vi "AmsRouterNotification Event Callback.vi"(4 "User Parameter":refnum<user-event>, 5 "Event Data":cluster{"sender":refnum<k24>, "e":refnum<k24>}, 6 "Control Ref":refnum<k24>, 7 "Event Common Data":T1) -> ()   [LabVIEW 2018, in "TwinCAT ADS.lvclass"]
uses:
  TwinCAT ADS.lvclass
  TwinCAT.Ads
  Controls/AMS Router Notification Event Data.ctl
  Controls/AMS Router State.ctl
  <vilib>/event_ctls.llb/usereventprio.ctl
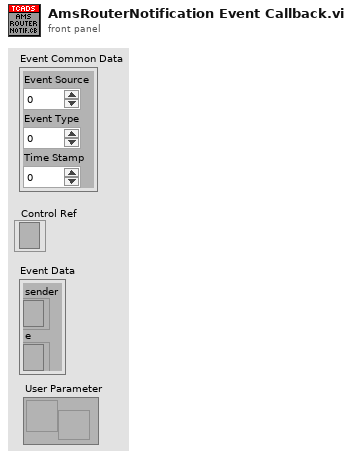
[diagram p1: front panel]
types:
  T1 = cluster{"Event Source":i32, "Event Type":u32, "Time Stamp":u32}
  T2 = typedef "usereventprio.ctl" = enum32{"high priority", "normal priority"}
  T3 = typedef "TwinCAT ADS.lvclass/AMS Router Notification Event Data.ctl" = cluster{"State":T4}
  T4 = typedef "TwinCAT ADS.lvclass/AMS Router State.ctl" = enum32{"Stop", "Start", "Removed", "Unknown"}
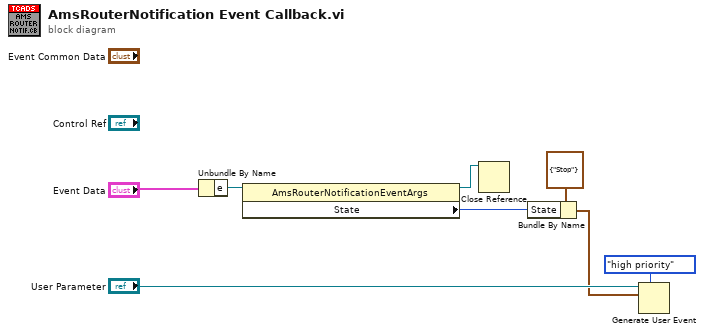
[diagram p0: block diagram]
diagram:
  n1 = Unbundle By Name("Event Data") -> ("e"=w7:refnum<k24>)
  n2 = property class="AmsRouterNotificationEventArgs"(reference=w7) -> (reference out=w6:refnum<k24>, "State"=w3:i32)  [unwired: 1 in, 1 out]
  n3 = Close Reference(reference=w6) -> ()  [unwired: 1 in, 1 out]
  n4 = Bundle By Name(cluster=T3 {"State"=enum."Stop"} ("event data"), "State"=w3) -> (w2:T3)
  n5 = Generate User Event(priority (normal)=usereventprio."high priority", user event="User Parameter", event data cluster=w2) -> ()  [unwired: 1 in, 2 out]
